vi "Segundos_String.vi"(1 "Total sec":dbl) -> (0 "TempsTotal":string)   [LabVIEW 2017]
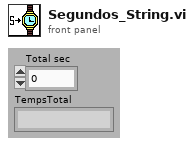
[diagram p1: front panel]
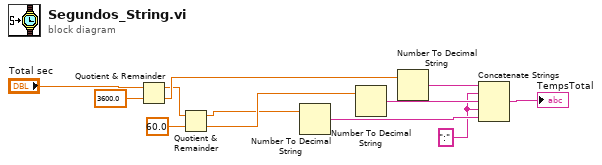
[diagram p0: block diagram]
diagram:
  w7 = ":" ("string")
  n1 = Quotient & Remainder(x="Total sec", y=3600.0) -> (x-y*floor(x/y)=w5:dbl, floor(x/y)=w6:dbl)
  n2 = Quotient & Remainder(x=w5, y=60.0) -> (x-y*floor(x/y)=w2:dbl, floor(x/y)=w3:dbl)
  n3 = Number To Decimal String(number=w2) -> (decimal integer string=w8:string)  [unwired: 1 in]
  n4 = Number To Decimal String(number=w3) -> (decimal integer string=w9:string)  [unwired: 1 in]
  n5 = Number To Decimal String(number=w6) -> (decimal integer string=w10:string)  [unwired: 1 in]
  n6 = Concatenate Strings(w10, w7, w9, w7, w8) -> (→"TempsTotal":string)
